vi "Get_Name_DoB.vi"(0 "Application_Directory":path, 11 "Error_In":errorcluster) -> (4 "Name_Out":string, 6 "DoB_Out":timestamp caption="DoB   :" format="%<%x>T", 15 "Error_Out":errorcluster)   [LabVIEW 2023]
doc: "This is a VI work as one of the front panel of the Game, asking the user their Name and Dob."
uses:
  Controls/Bool_Button.ctl
  Controls/State.ctl
panel:
  in  "Home":T1
  in  "Back?":T1
  in  "DoB":timestamp caption="DoB   :" format="%<%x>T"
  in  "Name":string caption="Name :"
  in  "Next?":T1
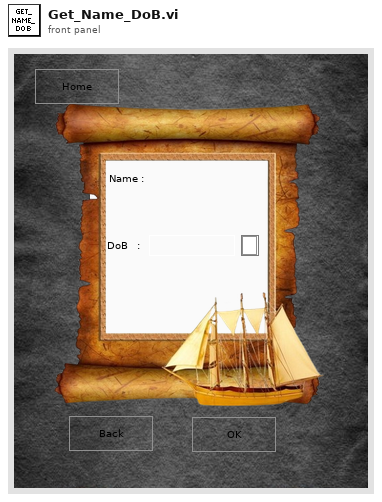
[diagram p1: front panel]
types:
  T1 = typedef "Bool_Button.ctl" = bool
  T2 = enum32{"Invalid", "Standard", "Closed", "Hidden", "Minimized", "Maximized"}
  T3 = typedef "State.ctl" = enum16{"Close", "Password_Popup", "Start_Popup", "Wizard_Msg", "Get_Name_DoB", "Lucky_Number", "Q-1", "Q-2", "Q-3", "Nature_of_the_Person"}
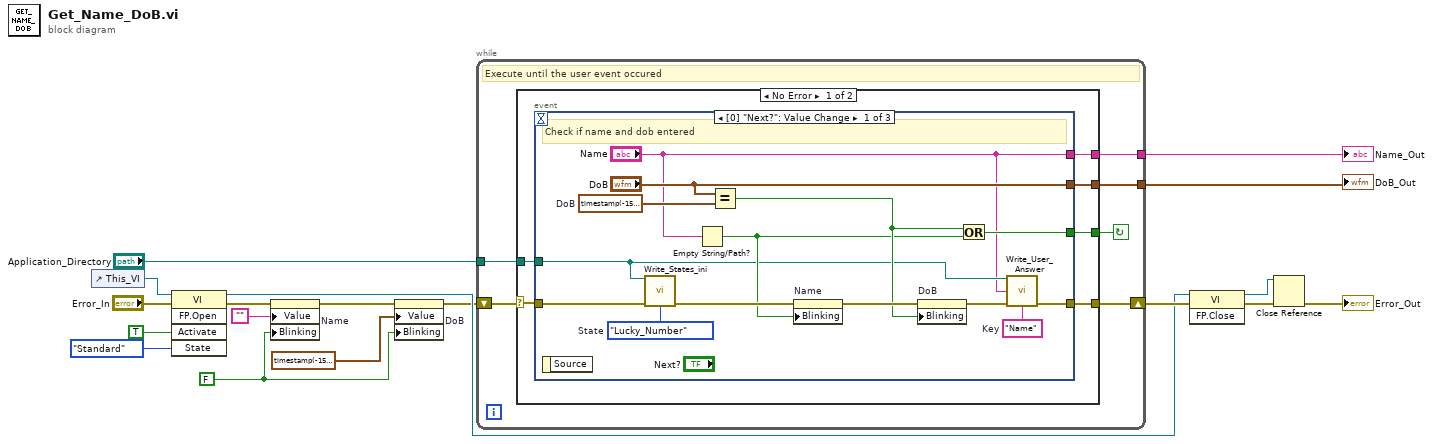
[diagram p0: block diagram]
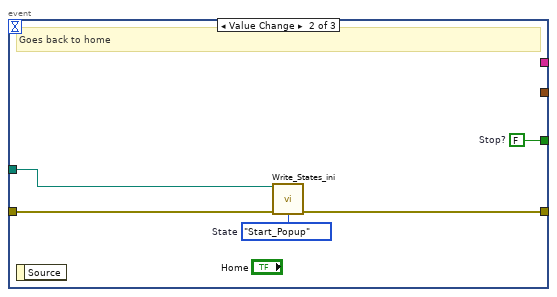
[diagram p2: hidden frame]
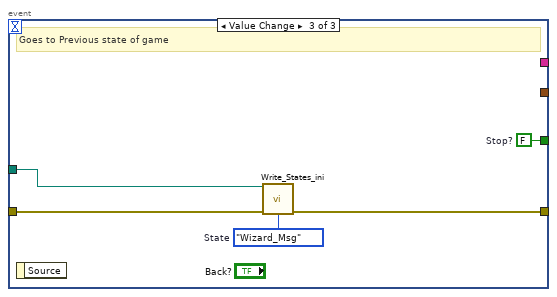
[diagram p3: hidden frame]
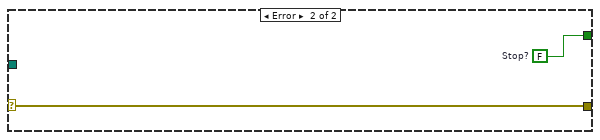
[diagram p4: hidden frame]
diagram:
  w4 = FALSE ("Blinking")
  n1 = control-ref of="This_VI"() -> (w15:refnum<vi>)
  n2 = invoke class="VI" method="FP.Open"(reference=w15, error in="Error_In", "Activate"=TRUE ("Activate?"), "State"=T2."Standard") -> (reference out=w10:refnum<vi>, error out=w14:errorcluster)  [unwired: 1 in, 3 out]
  n3 = property on="Name" class="Str"(error in=w14, "Value"="", "Blinking"=w4) -> (error out=w5:errorcluster)  [unwired: 1 in, 1 out]
  n4 = property on="DoB" class="AbsTime (strict)"(error in=w5, "Value"=timestamp(-157655308.61714554 s since 1904-01-01) ("DoB"), "Blinking"=w4) -> (error out=w6:errorcluster)  [unwired: 1 in, 1 out]
  n5 = while {
    shift-right: [w23] -> w11
    shift-left: w6 -> [w24]
    tunnel: [w22] -> w18
    tunnel: [w20] -> w17
    tunnel: "Application_Directory" -> [w19]
    stop <- w21 continue-if-true
    # "Execute until the user event occured"
    n6 = case shown="No Error" w24 {
      selector: w24 -> [w30 w56]
      tunnel: [w29 w56] -> w23
      tunnel: [w28 w55] -> w21
      tunnel: [w27 _] -> w22
      tunnel: [w26 _] -> w20
      tunnel: w19 -> [w25 _]
      frame No Error {
        n7 = event shown="[0] \"Next?\": Value Change" {
          selector: _ -> [_ _ _]
          dyn-events: _ -> [_ _ _]
          timeout: _ -> [_ _ _]
          tunnel: w30 -> [w43 w49 w54]
          tunnel: [w33 w48 w53] -> w29
          tunnel: [w44 w45 w50] -> w28
          tunnel: ["Name" _ _] -> w27
          tunnel: ["DoB" _ _] -> w26
          tunnel: w25 -> [w35 w46 w51]
          event Value Change {
            w31 = "Name"  # Key
            w36 = timestamp(-157655308.61714554 s since 1904-01-01)  # DoB
            w42 = State."Lucky_Number"  # State
            # "Check if name and dob entered"
            n8 = event-data() -> ()  [unwired: 1 in, 1 out]
            n9 = call "Write_States_ini.vi"("Application_Directory"=w35, "Error_In"=w43, "State"=w42) -> ("Error_Out"=w41:errorcluster)  [unwired: 12 in]
            n10 = Empty String/Path?(string/path="Name") -> (empty?=w38:bool)
            n11 = Equal?(x="DoB", y=w36) -> (x = y?=w39:bool)
            n12 = property on="Name" class="Str"(error in=w41, "Blinking"=w38) -> (error out=w40:errorcluster)  [unwired: 1 in, 1 out]
            n13 = property on="DoB" class="AbsTime (strict)"(error in=w40, "Blinking"=w39) -> (error out=w32:errorcluster)  [unwired: 1 in, 1 out]
            n14 = Or(x=w39, y=w38) -> (x .or. y?=w44:bool)
            n15 = call "Write_User_Answer.vi"("Application_Directory"=w35, "Data"="Name", "Error_In"=w32, "Key"=w31) -> ("Error_Out"=w33:errorcluster)  [unwired: 11 in]
          }
          event Value Change {
            w45 = FALSE  # Stop?
            w47 = State."Start_Popup"  # State
            # "Goes back to home"
            n16 = event-data() -> ()  [unwired: 1 in, 1 out]
            n17 = call "Write_States_ini.vi"("Application_Directory"=w46, "Error_In"=w49, "State"=w47) -> ("Error_Out"=w48:errorcluster)  [unwired: 12 in]
          }
          event Value Change {
            w50 = FALSE  # Stop?
            w52 = State."Wizard_Msg"  # State
            # "Goes to Previous state of game"
            n18 = event-data() -> ()  [unwired: 1 in, 1 out]
            n19 = call "Write_States_ini.vi"("Application_Directory"=w51, "Error_In"=w54, "State"=w52) -> ("Error_Out"=w53:errorcluster)  [unwired: 12 in]
          }
        }
      }
      frame Error {
        w55 = FALSE  # Stop?
      }
    }
  }
  "Name_Out" <- w18
  "DoB_Out" <- w17
  n20 = invoke class="VI" method="FP.Close"(reference=w10, error in=w11) -> (reference out=w7:refnum<vi>, error out=w9:errorcluster)  [unwired: 1 in, 1 out]
  n21 = Close Reference(reference=w7, error in (no error)=w9) -> (error out=→"Error_Out":errorcluster)
